vi "Test Missing VIs.vi"(11 "Test Case In":refnum<class "Missing in Project.lvclass">) -> (0 "error out":errorcluster, 3 "Test Case Out":refnum<class "Missing in Project.lvclass">)   [LabVIEW 2020, in "Missing in Project.lvclass"]
doc: "Tests to make sure all VIs and Ctls defined in the project are saved to disk."
uses:
  Missing in Project.lvclass
  C:/Program Files/National Instruments/LabVIEW 2024/vi.lib/Astemes/LUnit/Test Case.lvclass
  <vilib>/Astemes/LUnit/Test Case.lvclass/Test Case.ctl
  <vilib>/Astemes/LUnit/Append Pass Result.vi
  <vilib>/Astemes/LUnit/Append Fail Result.vi
  <vilib>/Astemes/LUnit/Run In UI.vi
  <vilib>/Utility/error.llb/Clear Errors.vi
  <vilib>/Astemes/LUnit/Test Case.lvclass
panel:
  out "Missing items":path[](array[path])
  out "Pass":bool
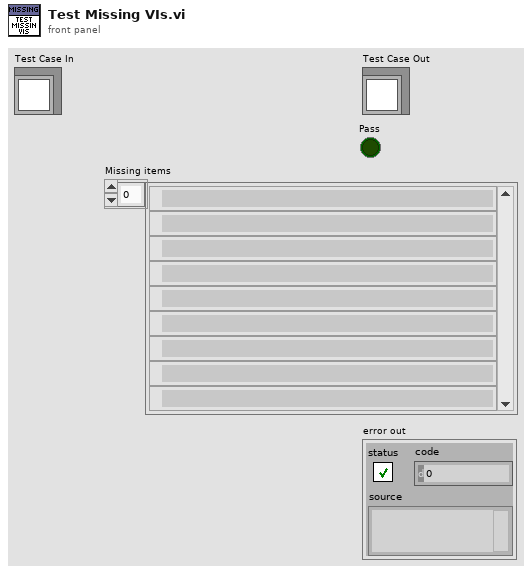
[diagram p1: front panel]
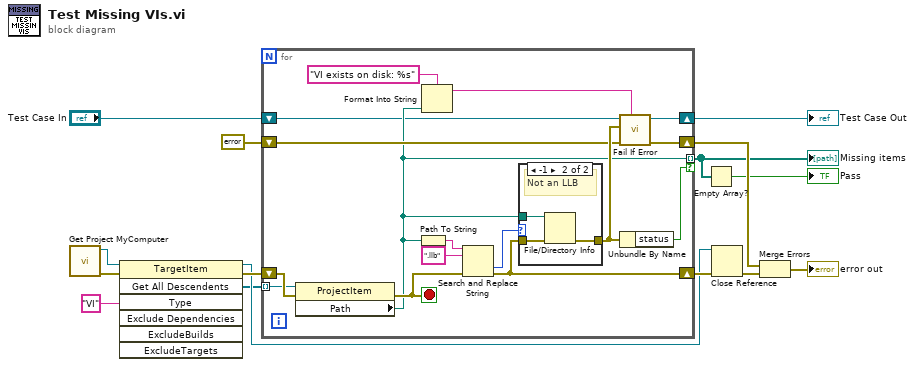
[diagram p0: block diagram]
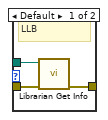
[diagram p2: hidden frame]
diagram:
  n1 = call "Get Project MyComputer.vi"() -> ("error out"=w9:errorcluster, "My Computer"=w1:refnum<vi>)  [unwired: 10 in]
  n2 = invoke on="Invoke Node" class="TargetItem" method="Get All Descendents"(reference=w1, error in=w9, "Type"="VI") -> (reference out=w8:refnum<vi>, error out=w15:errorcluster, "All Descendents"=w6:refnum<vi>[])  [unwired: 4 in, 4 out]
  n3 = for {
    tunnel: w6 -> [w25] mode=indexing
    shift-right: [w28] -> w14
    shift-left: w15 -> [w30]
    tunnel: [w20] -> w5 mode=indexing if=w24
    shift-right: [w27] -> w10
    shift-left: errorcluster {"status"=FALSE, "code"=0, "source"=""} ("error in (no error)") -> [w26]
    shift-right: [w17] -> w2
    shift-left: "Test Case In" -> [w18]
    stop <- w29 stop-if-true
    n4 = property on="Property Node" class="ProjectItem"(reference=w25, error in=w30) -> (error out=w29:errorcluster, "Path"=w20:path)  [unwired: 1 out]
    n5 = Path To String(path=w20) -> (string=w23:string)
    n6 = Format Into String(format string="VI exists on disk: %s" ("Label"), w20) -> (resulting string=w19:string)  [unwired: 2 in, 1 out]
    n7 = Search and Replace String(input string=w23, search string=".llb", error in=w29) -> (offset past replacement=w21:i32, error out=w28:errorcluster)  [unwired: 5 in, 2 out]
    n8 = case shown="-1" w21 {
      tunnel: w28 -> [w34 w37]
      tunnel: [w33 w36] -> w31
      tunnel: w20 -> [w32 w35]
      frame Default {
        # "LLB"
        n9 = call <vilib>:"Librarian Get Info.vi"("error in (no error)"=w34, "path"=w32) -> ("error out"=w33:errorcluster)  [unwired: 7 in, 2 out]
      }
      frame -1 {
        # "Not an LLB"
        n10 = File/Directory Info(path=w35, error in=w37) -> (error out=w36:errorcluster)  [unwired: 6 out]
      }
    }
    n11 = call <vilib>:"Fail If Error.vi"("Description"=w19, "error in (no error)"=w26, "Assert error"=w31, "LUnit Test Case In"=w18) -> ("error out"=w27:errorcluster, "LUnit Test Case Out"=w17:refnum<class "Missing in Project.lvclass">)  [unwired: 6 in]
    n12 = Unbundle By Name(w31) -> ("status"=w24:bool)
  }
  "Missing items" <- w5
  "Test Case Out" <- w2
  n13 = Empty Array?(array=w5) -> (empty?=→"Pass":bool)
  n14 = Close Reference(reference=w8, error in (no error)=w14) -> (error out=w13:errorcluster)
  n15 = Merge Errors(w10, w13) -> (→"error out":errorcluster)
